vi "ETH_11 Main.vi"(8 "error in":errorcluster, 10 "data in":string, 11 "ETH11-Q":refnum<queue>) -> (0 "error out":errorcluster)   [LabVIEW 2022 SP3]
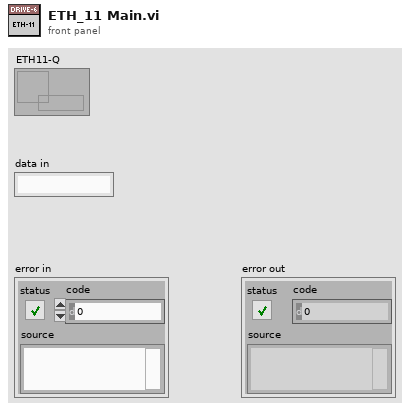
[diagram p1: front panel]
types:
  T1 = cluster{"Run ACK":dbl, "Frequency":dbl, "Speed":dbl, "RPM Dir":dbl, "VDC":dbl, "IDC":dbl, "Movable IDC":dbl, "M-State":dbl}
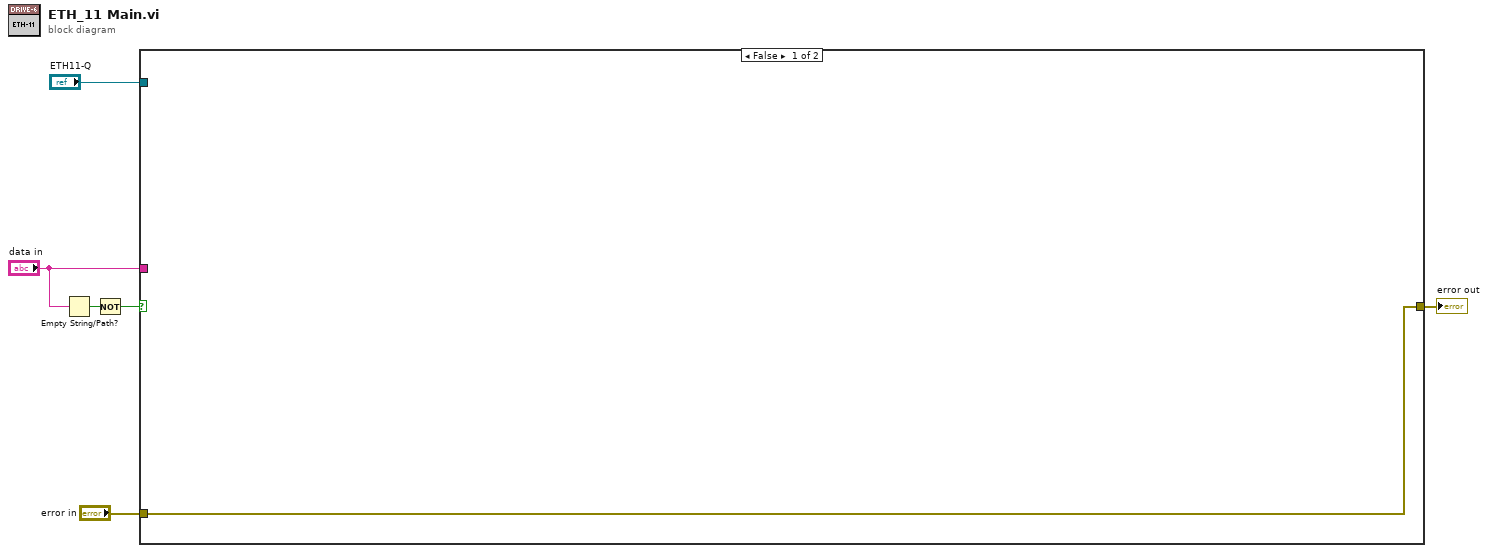
[diagram p0: block diagram]
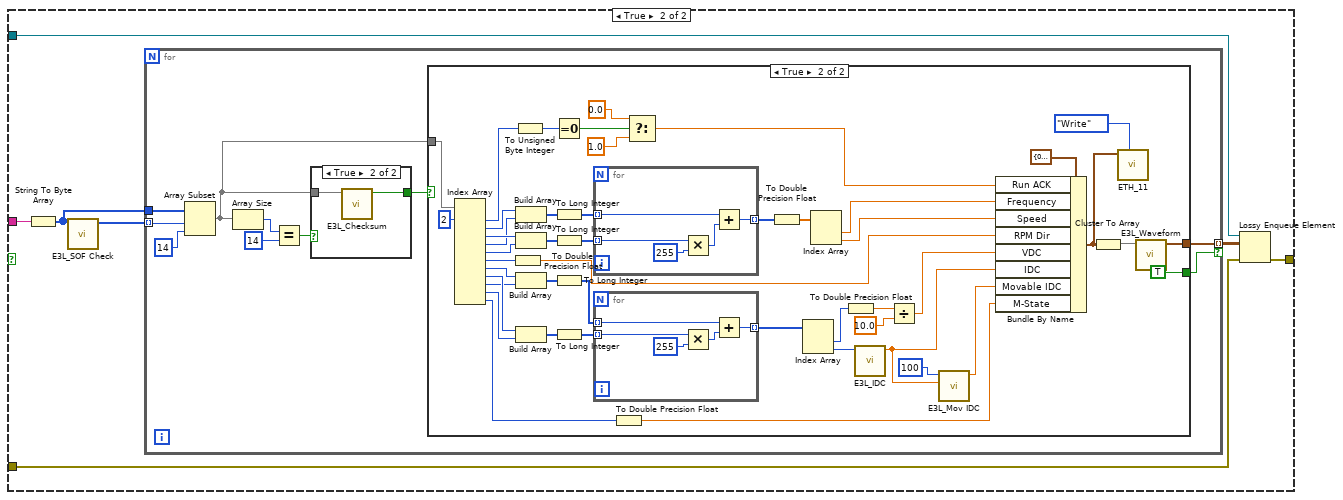
[diagram p2: hidden frame]
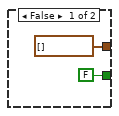
[diagram p3: hidden frame]
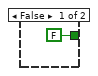
[diagram p4: hidden frame]
diagram:
  n1 = Empty String/Path?(string/path="data in") -> (empty?=w6:bool)
  n2 = Not(x=w6) -> (.not. x?=w5:bool)
  n3 = case shown="False" w5 {
    tunnel: "data in" -> [_ w14]
    tunnel: "ETH11-Q" -> [_ w10]
    tunnel: "error in" -> [w7 w9]
    tunnel: [w7 w8] -> w1
    frame False {
    }
    frame True {
      n4 = String To Byte Array(string=w14) -> (unsigned byte array=w12:u8[])
      n5 = call "E3L_SOF Check.vi"("Bytes data in"=w12) -> ("index of passed smpl"=w13:i32[])  [unwired: 8 in, 2 out]
      n6 = for {
        tunnel: w13 -> [w21] mode=indexing
        tunnel: w12 -> [w20]
        tunnel: [w16] -> w11 mode=indexing if=w15
        n7 = Array Subset(array=w20, index=w21, length=14) -> (w17:u8[])
        n8 = Array Size(array=w17) -> (size(s)=w23:i32)
        n9 = Equal?(x=w23, y=14) -> (x = y?=w19:bool)
        n10 = case shown="True" w19 {
          tunnel: w17 -> [_ w86]
          tunnel: [FALSE ("Checksum") w85] -> w18
          frame False {
          }
          frame True {
            n11 = call "E3L_Checksum.vi"("Data"=w86) -> ("Checksum"=w85:bool)  [unwired: 10 in]
          }
        }
        n12 = case shown="True" w18 {
          tunnel: w17 -> [_ w49]
          tunnel: [waveform(dbl)[] [] ("WF out") w30] -> w16
          tunnel: [FALSE TRUE] -> w15
          frame False {
          }
          frame True {
            n13 = Index Array(array=w49, index #1=2 ("index")) -> (element #1=w71:u8, element #2=w65:u8, element #3=w64:u8, element #4=w63:u8, element #5=w62:u8, element #6=w60:u8, element #7=w55:u8, element #8=w54:u8, element #9=w53:u8, element #10=w52:u8, element #11=w48:u8)  [unwired: 10 in]
            n14 = To Double Precision Float(number=w60) -> (double precision float=w39:dbl)
            n15 = To Unsigned Byte Integer(number=w71) -> (unsigned 8bit integer=w72:u8)
            n16 = Build Array(w65, w63) -> (w70:u8[])
            n17 = Build Array(w64, w62) -> (w69:u8[])
            n18 = Build Array(w55, w53) -> (w59:u8[])
            n19 = Build Array(w54, w52) -> (w58:u8[])
            n20 = Equal To 0?(x=w72) -> (x = 0?=w73:bool)
            n21 = To Long Integer(number=w70) -> (32bit integer=w67:i32[])
            n22 = To Long Integer(number=w69) -> (32bit integer=w66:i32[])
            n23 = To Long Integer(number=w59) -> (32bit integer=w57:i32[])
            n24 = To Long Integer(number=w58) -> (32bit integer=w56:i32[])
            n25 = for {
              tunnel: w67 -> [w83] mode=indexing
              tunnel: w66 -> [w82] mode=indexing
              tunnel: [w80] -> w68 mode=indexing
              n26 = Multiply(x=w82, y=255) -> (x*y=w81:i32)
              n27 = Add(x=w83, y=w81) -> (x+y=w80:i32)
            }
            n28 = for {
              tunnel: w57 -> [w78] mode=indexing
              tunnel: w56 -> [w77] mode=indexing
              tunnel: [w75] -> w37 mode=indexing
              n29 = Multiply(x=w77, y=255) -> (x*y=w76:i32)
              n30 = Add(x=w78, y=w76) -> (x+y=w75:i32)
            }
            n31 = To Double Precision Float(number=w48) -> (double precision float=w32:dbl)
            n32 = Select(t=0.0, s=w73, f=1.0) -> (s? t:f=w45:dbl)
            n33 = To Double Precision Float(number=w68) -> (double precision float=w61:dbl[])
            n34 = Index Array(array=w37) -> (element #1=w41:i32, element #2=w36:i32)  [unwired: 2 in]
            n35 = Index Array(array=w61) -> (element #1=w44:dbl, element #2=w40:dbl)  [unwired: 2 in]
            n36 = To Double Precision Float(number=w41) -> (double precision float=w43:dbl)
            n37 = call "E3L_IDC.vi"("IDC in"=w36) -> ("IDC out"=w35:dbl)  [unwired: 10 in]
            n38 = Divide(x=w43, y=10.0) -> (x/y=w38:dbl)
            n39 = call "E3L_Mov IDC.vi"("Idc"=w35, "SampleSize"=100) -> ("Mean"=w33:dbl)  [unwired: 9 in]
            n40 = Bundle By Name(cluster=T1 {"Run ACK"=0.0, "Frequency"=0.0, "Speed"=0.0, "RPM Dir"=0.0, "VDC"=0.0, "IDC"=0.0, "Movable IDC"=0.0, "M-State"=0.0} ("output cluster"), "Run ACK"=w45, "Frequency"=w44, "Speed"=w40, "RPM Dir"=w39, "VDC"=w38, "IDC"=w35, "Movable IDC"=w33, "M-State"=w32) -> (w27:T1)
            n41 = Cluster To Array(cluster=w27) -> (array=w31:dbl[])
            n42 = call "ETH_11.vi"("Enum"=enum16{"Read", "Write"}."Write", "ETH 11"=w27) -> ()  [unwired: 8 in, 2 out]
            n43 = call "E3L_Waveform.vi"("Data in"=w31) -> ("WF out"=w30:waveform(dbl)[])  [unwired: 10 in]
          }
        }
      }
      n44 = Lossy Enqueue Element(queue=w10, element=w11, error in (no error)=w9) -> (error out=w8:errorcluster)  [unwired: 3 out]
    }
  }
  "error out" <- w1
